vi "Open_Drive_PIDFs.vi"() -> (0 "Left F":dbl, 3 "Right_F":dbl, 4 "Left D":dbl, 5 "Right_D":dbl, 6 "Left I":dbl, 7 "Right_I":dbl, 8 "Left P":dbl, 11 "Right_P":dbl=1.0)   [LabVIEW 2019]
uses:
  <vilib>/Utility/file.llb/Read Delimited Spreadsheet (string).vi
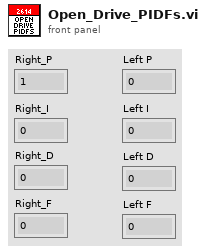
[diagram p1: front panel]
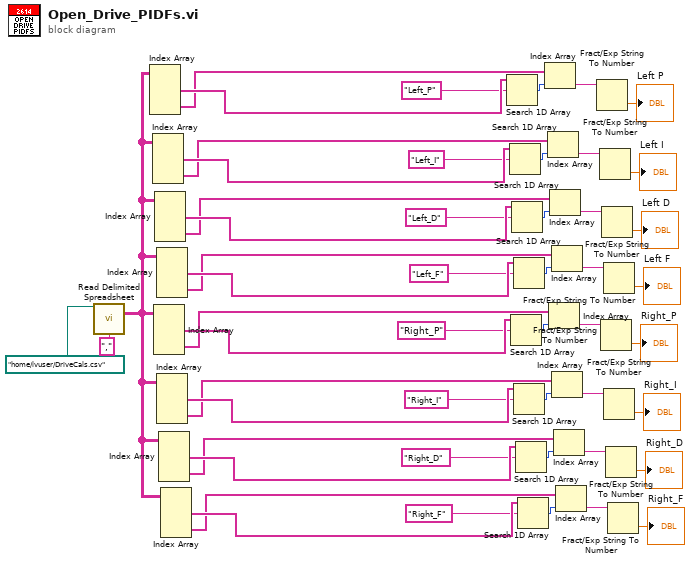
[diagram p0: block diagram]
diagram:
  n1 = call-poly <vilib>:"Read Delimited Spreadsheet.vi"("file path (dialog if empty)"=path "/home/lvuser/DriveCals.csv", "delimiter (\\t)"="," ("delimiter (\\t)")) -> ("all rows"=w1:string[][])  [unwired: 8 in, 5 out]
  n2 = Index Array(array=w1) -> (element #1=w25:string[], element #2=w24:string[])  [unwired: 4 in]
  n3 = Index Array(array=w1) -> (element #1=w19:string[], element #2=w18:string[])  [unwired: 4 in]
  n4 = Index Array(array=w1) -> (element #1=w49:string[], element #2=w48:string[])  [unwired: 4 in]
  n5 = Index Array(array=w1) -> (element #1=w13:string[], element #2=w12:string[])  [unwired: 4 in]
  n6 = Index Array(array=w1) -> (element #1=w7:string[], element #2=w6:string[])  [unwired: 4 in]
  n7 = Index Array(array=w1) -> (element #1=w43:string[], element #2=w42:string[])  [unwired: 4 in]
  n8 = Index Array(array=w1) -> (element #1=w37:string[], element #2=w36:string[])  [unwired: 4 in]
  n9 = Index Array(array=w1) -> (element #1=w31:string[], element #2=w30:string[])  [unwired: 4 in]
  n10 = Search 1D Array(1D array=w25, element="Left_P") -> (index of element=w23:i32)  [unwired: 1 in]
  n11 = Search 1D Array(1D array=w19, element="Left_I") -> (index of element=w17:i32)  [unwired: 1 in]
  n12 = Search 1D Array(1D array=w49, element="Right_P") -> (index of element=w47:i32)  [unwired: 1 in]
  n13 = Search 1D Array(1D array=w13, element="Left_D") -> (index of element=w11:i32)  [unwired: 1 in]
  n14 = Search 1D Array(1D array=w7, element="Left_F") -> (index of element=w5:i32)  [unwired: 1 in]
  n15 = Search 1D Array(1D array=w43, element="Right_I") -> (index of element=w41:i32)  [unwired: 1 in]
  n16 = Search 1D Array(1D array=w37, element="Right_D") -> (index of element=w35:i32)  [unwired: 1 in]
  n17 = Search 1D Array(1D array=w31, element="Right_F") -> (index of element=w29:i32)  [unwired: 1 in]
  n18 = Index Array(array=w24, index=w23) -> (element=w21:string)
  n19 = Index Array(array=w18, index=w17) -> (element=w15:string)
  n20 = Index Array(array=w48, index=w47) -> (element=w45:string)
  n21 = Index Array(array=w12, index=w11) -> (element=w9:string)
  n22 = Index Array(array=w6, index=w5) -> (element=w3:string)
  n23 = Index Array(array=w42, index=w41) -> (element=w39:string)
  n24 = Index Array(array=w36, index=w35) -> (element=w33:string)
  n25 = Index Array(array=w30, index=w29) -> (element=w27:string)
  n26 = Fract/Exp String To Number(string=w21) -> (number=→"Left P":dbl)  [unwired: 3 in, 1 out]
  n27 = Fract/Exp String To Number(string=w15) -> (number=→"Left I":dbl)  [unwired: 3 in, 1 out]
  n28 = Fract/Exp String To Number(string=w45) -> (number=→"Right_P":dbl)  [unwired: 3 in, 1 out]
  n29 = Fract/Exp String To Number(string=w9) -> (number=→"Left D":dbl)  [unwired: 3 in, 1 out]
  n30 = Fract/Exp String To Number(string=w3) -> (number=→"Left F":dbl)  [unwired: 3 in, 1 out]
  n31 = Fract/Exp String To Number(string=w39) -> (number=→"Right_I":dbl)  [unwired: 3 in, 1 out]
  n32 = Fract/Exp String To Number(string=w33) -> (number=→"Right_D":dbl)  [unwired: 3 in, 1 out]
  n33 = Fract/Exp String To Number(string=w27) -> (number=→"Right_F":dbl)  [unwired: 3 in, 1 out]
